vi "Set Data Binding.vi"(8 "error in (no error)":errorcluster, 11 "DataGridView in":refnum<class "DataGridView.lvclass">) -> (0 "error out":errorcluster, 3 "DataGridView out":refnum<class "DataGridView.lvclass">)   [LabVIEW 2014, in "DataGridView.lvclass"]
doc: "This is a simple data binding step that connects the dataTable with all the data in it, into the DataGridView for display. The columns get bound and autogenerated by the datagridview for any object types with native support in this step. The next step is to set any custom column types to define specific object types."
uses:
  DataGridView.lvclass
  DataGridView.lvclass/DataGridView.ctl
  System.Windows.Forms
  Read DataGridView.vi
  System.Data
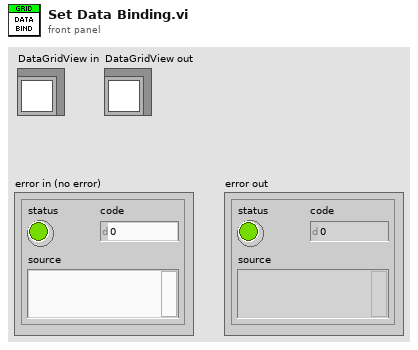
[diagram p1: front panel]
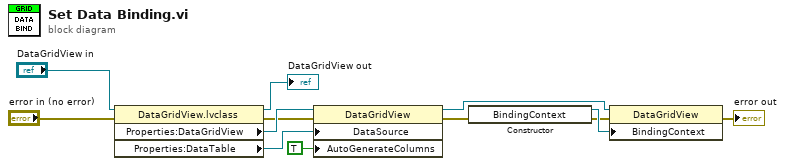
[diagram p0: block diagram]
diagram:
  n1 = property class="DataGridView.lvclass"(reference="DataGridView in", error in="error in (no error)") -> (reference out=→"DataGridView out":refnum<class "DataGridView.lvclass">, error out=w2:errorcluster, "Properties:DataGridView"=w6:refnum<k24>, "Properties:DataTable"=w5:refnum<k24>)
  n2 = property class="DataGridView"(reference=w6, error in=w2, "DataSource"=w5, "AutoGenerateColumns"=TRUE) -> (reference out=w10:refnum<k24>, error out=w12:errorcluster)
  n3 = constructor class="BindingContext"(error in=w12) -> (reference out=w9:refnum<k24>, error out=w8:errorcluster)  [unwired: 2 in, 1 out]
  n4 = property class="DataGridView"(reference=w10, error in=w8, "BindingContext"=w9) -> (error out=→"error out":errorcluster)  [unwired: 1 out]
